vi "P9_bis.vi"() -> ()   [LabVIEW 2018]
uses:
  <vilib>/vision/NI_Vision_Development_Module.lvlib
panel:
  in  "stop":bool
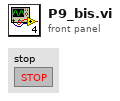
[diagram p1: front panel]
types:
  T1 = typedef "Image Type" = u32
  T2 = typedef "IMAQ Image.ctl" = refnum<image>
  T3 = cluster{"Browser Size":cluster{"X":i32, "Y":i32}, "Images per Line":i32, "Background Color":u32, "Frame Size":i32, "Frame Style":enum16{"Raised", "Bevelled", "Outline", "Hidden", "Step", "Raised Outline"}}
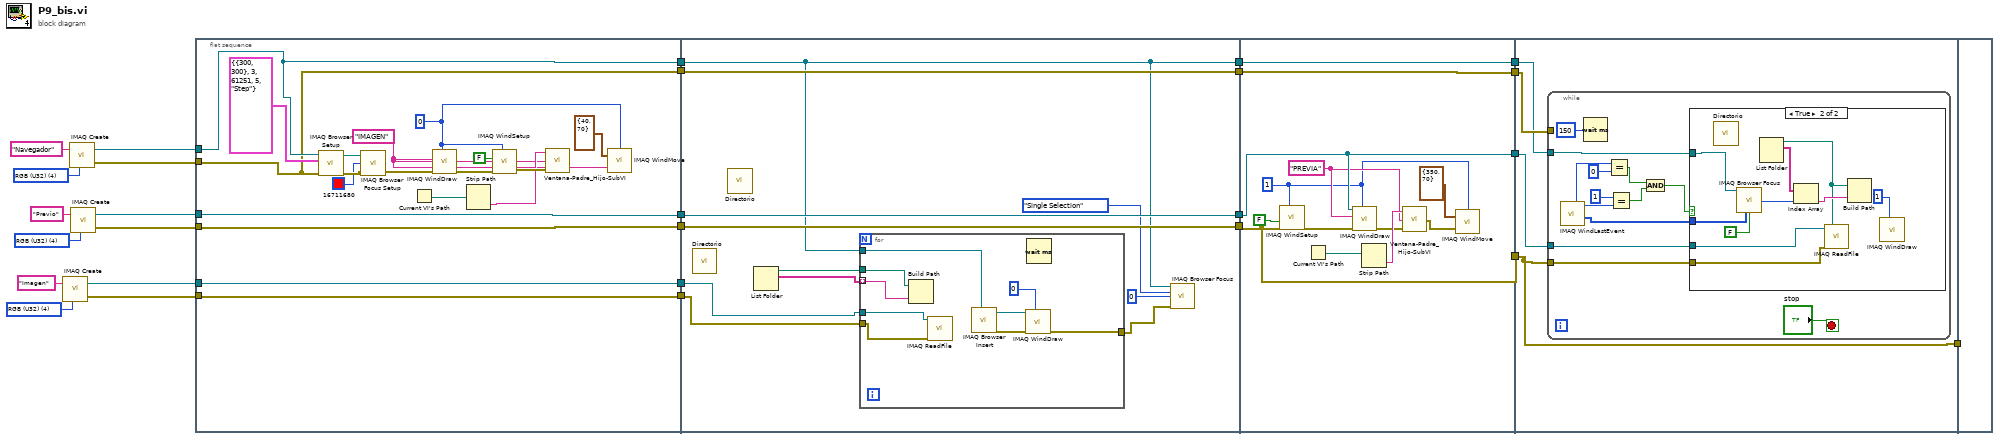
[diagram p0: block diagram]
diagram:
  w22 = T1 4 items=["Grayscale (U8)", "Grayscale (I16)", "Grayscale (SGL)", "Complex (CSG)", "RGB (U32)", "HSL (U32)", "RGB (U64)", "Grayscale (U16)"] ("Image Type")
  w24 = T1 4 items=["Grayscale (U8)", "Grayscale (I16)", "Grayscale (SGL)", "Complex (CSG)", "RGB (U32)", "HSL (U32)", "RGB (U64)", "Grayscale (U16)"] ("Image Type")
  w26 = T1 4 items=["Grayscale (U8)", "Grayscale (I16)", "Grayscale (SGL)", "Complex (CSG)", "RGB (U32)", "HSL (U32)", "RGB (U64)", "Grayscale (U16)"] ("Image Type")
  n1 = call "IMAQ Create"("Image Name"="Imagen", "Image Type"=w22) -> ("New Image"=w21:T2, "error out"=w20:errorcluster)  [unwired: 3 in]
  n2 = call "IMAQ Create"("Image Name"="Navegador", "Image Type"=w26) -> ("New Image"=w16:T2, "error out"=w17:errorcluster)  [unwired: 3 in]
  n3 = call "IMAQ Create"("Image Name"="Previo", "Image Type"=w24) -> ("New Image"=w18:T2, "error out"=w19:errorcluster)  [unwired: 3 in]
  n4 = flat-sequence {
    tunnel: w21 -> [w44]
    tunnel: w20 -> [w43]
    tunnel: w19 -> [w45]
    tunnel: w18 -> [w46]
    tunnel: w17 -> [w40]
    tunnel: w16 -> [w41]
    tunnel: [w46] -> w15
    tunnel: [w45] -> w14
    tunnel: [w44] -> w13
    tunnel: [w43] -> w12
    tunnel: [w41] -> w11
    tunnel: [w40] -> w10
    tunnel: w15 -> [w52]
    tunnel: w14 -> [w51]
    tunnel: w13 -> [w55]
    tunnel: w12 -> [w54]
    tunnel: w11 -> [w50]
    tunnel: w10 -> [w53]
    tunnel: [w50] -> w9
    tunnel: [w53] -> w8
    tunnel: [w52] -> w7
    tunnel: [w51] -> w6
    tunnel: w9 -> [w75]
    tunnel: w8 -> [w74]
    tunnel: w7 -> [w76]
    tunnel: w6 -> [w78]
    tunnel: [w76] -> w5
    tunnel: [w78] -> w4
    tunnel: [w75] -> w3
    tunnel: [w74] -> w2
    tunnel: w5 -> [w82]
    tunnel: w4 -> [w83]
    tunnel: w3 -> [w80]
    tunnel: w2 -> [w81]
    tunnel: [w83] -> w1
    tunnel: w1 -> [_]
    frame #0 {
      w29 = 0 ("Window Number (0...15)")
      w28 = "IMAGEN" ("Title")
      n5 = call "IMAQ Browser Setup"("error in (no error)"=w40, "Browser Info"=T3 {"Browser Size"={"X"=300, "Y"=300}, "Images per Line"=3, "Background Color"=61251, "Frame Size"=5, "Frame Style"=enum."Step"}, "Image In"=w41) -> ("error out"=w38:errorcluster, "Image Browser Out"=w39:T2)  [unwired: 1 in, 2 out]
      n6 = call "IMAQ Browser Focus Setup"("error in (no error)"=w38, "Focus Color"=u32 16711680, "Image Browser In"=w39) -> ("error out"=w36:errorcluster)  [unwired: 1 in, 1 out]
      n7 = Current VI's Path() -> (path=w32:path)
      n8 = call "IMAQ WindDraw"("Window Number (0...15)"=w29, "error in (no error)"=w36, "Title"=w28) -> ("error out"=w35:errorcluster)  [unwired: 7 in, 1 out]
      n9 = Strip Path(path=w32) -> (name=w31:string)  [unwired: 1 out]
      n10 = call "IMAQ WindSetup"("Window Number (0...15)"=w29, "error in (no error)"=w35, "Window can close? (Yes)"=FALSE) -> ("error out"=w33:errorcluster)  [unwired: 8 in]
      n11 = call "Ventana-Padre_Hijo-SubVI.vi"("error out"=w28, "error in (no error)"=w33, "Child Window Name"=w28, "Parent Window Name"=w31) -> ()
      n12 = call "IMAQ WindMove"("Window Number (0...15)"=w29, "Coordinates (screen)"=cluster{"X Position":i32, "Y Position":i32} {"X Position"=40, "Y Position"=70}, "error in (no error)"=w28) -> ()  [unwired: 2 in, 2 out]
    }
    frame #1 {
      n13 = call "Directorio.vi"() -> ()  [unwired: 12 in]
      n14 = call "Directorio.vi"() -> ()  [unwired: 12 in]
      n15 = List Folder() -> (path out=w57:path, filenames=w56:string[])  [unwired: 4 in, 2 out]
      n16 = for {
        tunnel: w57 -> [w66]
        tunnel: w56 -> [w65] mode=indexing
        tunnel: w55 -> [w64]
        tunnel: w54 -> [w63]
        tunnel: w50 -> [w62]
        tunnel: [w58] -> w47
        n17 = Build Path(base path=w66, name or relative path=w65) -> ()  [unwired: 1 out]
        n18 = call <userlib>:"IMAQ ReadFile.vi"("error in (no error)"=w63, "Image"=w64) -> ()  [unwired: 5 in, 5 out]
        n19 = call "IMAQ Browser Insert"("Image Browser In"=w62) -> ("error out"=w59:errorcluster, "Image Browser Out"=w60:T2)  [unwired: 6 in, 3 out]
        n20 = call "IMAQ WindDraw"("Window Number (0...15)"=0, "error in (no error)"=w59, "Image"=w60) -> ("error out"=w58:errorcluster)  [unwired: 7 in, 1 out]
        n21 = Wait (ms)() -> ()  [unwired: 1 in, 1 out]
      }
      n22 = call "IMAQ Browser Focus"("Image Browser In"=w50, "Selection Mode"=enum16{"Single Selection", "Multiple Selection"}."Single Selection", "Index"=0, "error in (no error)"=w47) -> ()  [unwired: 6 in, 6 out]
    }
    frame #2 {
      w71 = "PREVIA" ("Title")
      w68 = 1 ("Window Number (0...15)")
      n23 = call "IMAQ WindSetup"("Window Number (0...15)"=w68, "error in (no error)"=w78, "Window has title bar? (Yes)"=FALSE) -> ("error out"=w77:errorcluster)  [unwired: 8 in]
      n24 = Current VI's Path() -> (path=w73:path)
      n25 = call "IMAQ WindDraw"("Window Number (0...15)"=w68, "error in (no error)"=w77, "Title"=w71, "Image"=w76) -> ("error out"=w70:errorcluster)  [unwired: 6 in, 1 out]
      n26 = Strip Path(path=w73) -> (name=w72:string)  [unwired: 1 out]
      n27 = call "Ventana-Padre_Hijo-SubVI.vi"("error in (no error)"=w70, "Child Window Name"=w71, "Parent Window Name"=w72) -> ("error out"=w67:errorcluster)
      n28 = call "IMAQ WindMove"("Window Number (0...15)"=w68, "Coordinates (screen)"=cluster{"X Position":i32, "Y Position":i32} {"X Position"=350, "Y Position"=70}, "error in (no error)"=w67) -> ()  [unwired: 2 in, 2 out]
    }
    frame #3 {
      n29 = while {
        tunnel: w83 -> [w93]
        tunnel: w82 -> [w94]
        tunnel: w81 -> [_]
        tunnel: w80 -> [w91]
        stop <- "stop" stop-if-true
        n30 = call "IMAQ WindLastEvent"() -> ("Coordinates"=w95:i32[], "Event"=w90:i32, "Window Number (0...15)"=w88:i32)  [unwired: 6 in, 3 out]
        n31 = Wait (ms)(milliseconds to wait=u32 150) -> ()  [unwired: 1 out]
        n32 = Equal?(x=w88, y=0) -> (x = y?=w86:bool)
        n33 = Equal?(x=1, y=w90) -> (x = y?=w85:bool)
        n34 = And(x=w86, y=w85) -> (x .and. y?=w84:bool)
        n35 = case shown="True" w84 {
          tunnel: w95 -> [_ w106]
          tunnel: w94 -> [_ w100]
          tunnel: w93 -> [_ w99]
          tunnel: w91 -> [_ w104]
          frame False {
          }
          frame True {
            n36 = call "Directorio.vi"() -> ()  [unwired: 12 in]
            n37 = call "IMAQ Browser Focus"("Image Browser In"=w104, "Pixel Position"=w106, "Get/Set (Set)"=FALSE) -> ("Index Out"=w103:i32)  [unwired: 7 in, 5 out]
            n38 = List Folder() -> (path out=w98:path, filenames=w102:string[])  [unwired: 4 in, 2 out]
            n39 = Index Array(array=w102, index=w103) -> (element=w101:string)
            n40 = call <userlib>:"IMAQ ReadFile.vi"("File Path"=w98, "error in (no error)"=w99, "Image"=w100) -> ()  [unwired: 4 in, 5 out]
            n41 = Build Path(base path=w98, name or relative path=w101) -> ()  [unwired: 1 out]
            n42 = call "IMAQ WindDraw"("Window Number (0...15)"=1) -> ()  [unwired: 9 in, 2 out]
          }
        }
      }
    }
    frame #4 {
    }
  }
